vi "Close.vi"(8 "error in (no error)":errorcluster, 11 "StringReader in":refnum<class "StringReader.lvclass">) -> (0 "error out":errorcluster, 3 "StringReader out":refnum<class "StringReader.lvclass">)   [LabVIEW 2013, in "StringReader.lvclass"]
doc: "Closes all open references and reserved resources for the reader"
uses:
  StringReader.lvclass
  BaseReader/BaseReader.lvclass
  StringReader.lvclass/StringReader.ctl
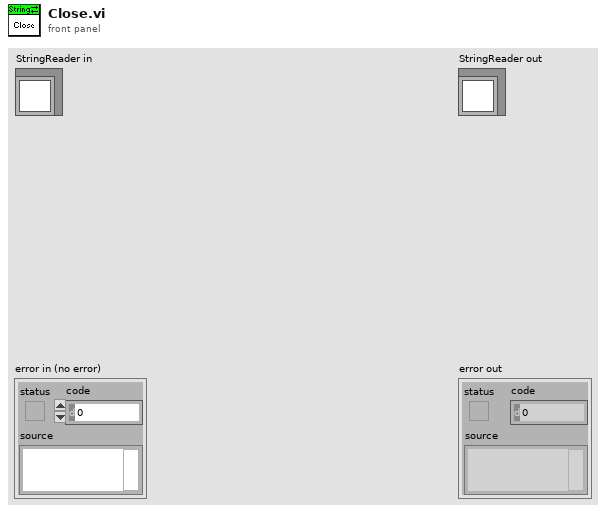
[diagram p1: front panel]
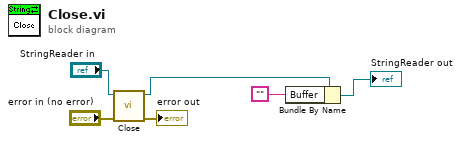
[diagram p0: block diagram]
diagram:
  n1 = call-parent "Close.vi"("error in (no error)"="error in (no error)", "BaseReader in"="StringReader in") -> ("error out"=→"error out":errorcluster, "BaseReader out"=w3:refnum<class "StringReader.lvclass">)  [unwired: 8 in]
  n2 = Bundle By Name(cluster=w3, "Buffer"="" ("Empty String Constant")) -> (→"StringReader out":refnum<class "StringReader.lvclass">)
